vi "Time.vi"(8 "error in (no error)":errorcluster, 10 "Control In":T1={"I-O.lvclass"=refnum, "Gantry"=refnum, "Dispenser"="COM1"}, 11 "C4 Dispense in":refnum<class "Iterative Dispense.lvclass">) -> (0 "error out":errorcluster, 1 "Timing Data":i32[](array[numeric]), 2 "Control Out":T1={"I-O.lvclass"=refnum, "Gantry"=refnum, "Dispenser"="COM1"}, 3 "C4 Dispense out":refnum<class "Iterative Dispense.lvclass">)   [LabVIEW 2020, in "Iterative Dispense.lvclass"]
uses:
  Iterative Dispense.lvclass
  C:/Users/HEP/Documents/GitHub/UCSB-Gantry-HEP/Classes/Routine/Dispense/Dispense.lvclass
  Controller/Controllers.ctl
  Controller/I-O/I-O.lvclass
  C:/Program Files (x86)/Aerotech/A3200/LabVIEW/2010/Bin/Aerotech.A3200.dll
  Program Files (x86)/Aerotech/A3200/LabVIEW/2010/Bin/Aerotech.A3200.dll
  Iterative Dispense.lvclass/Iterative Dispense.ctl
  Controller/Motion/Motion.lvclass
  Controller/Motion/A3200/A3200.lvclass
  Controller/Controller.lvclass
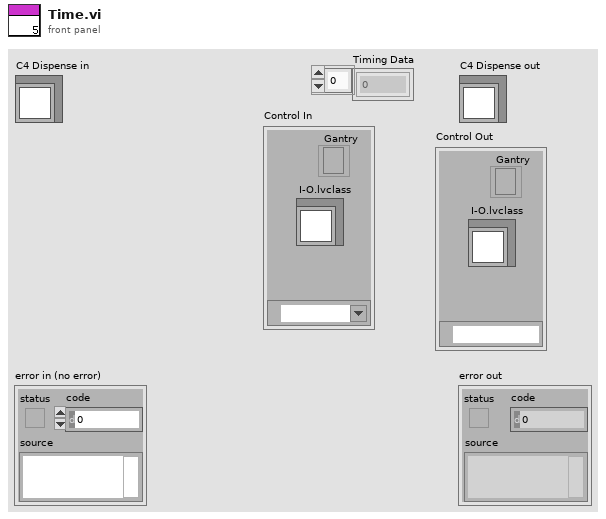
[diagram p1: front panel]
types:
  T1 = typedef "Controller.lvclass/Controllers.ctl" = cluster{"I-O.lvclass":refnum<class "I-O.lvclass">, "Gantry":refnum<k24>, "Dispenser":refnum<visa-resource-name>}
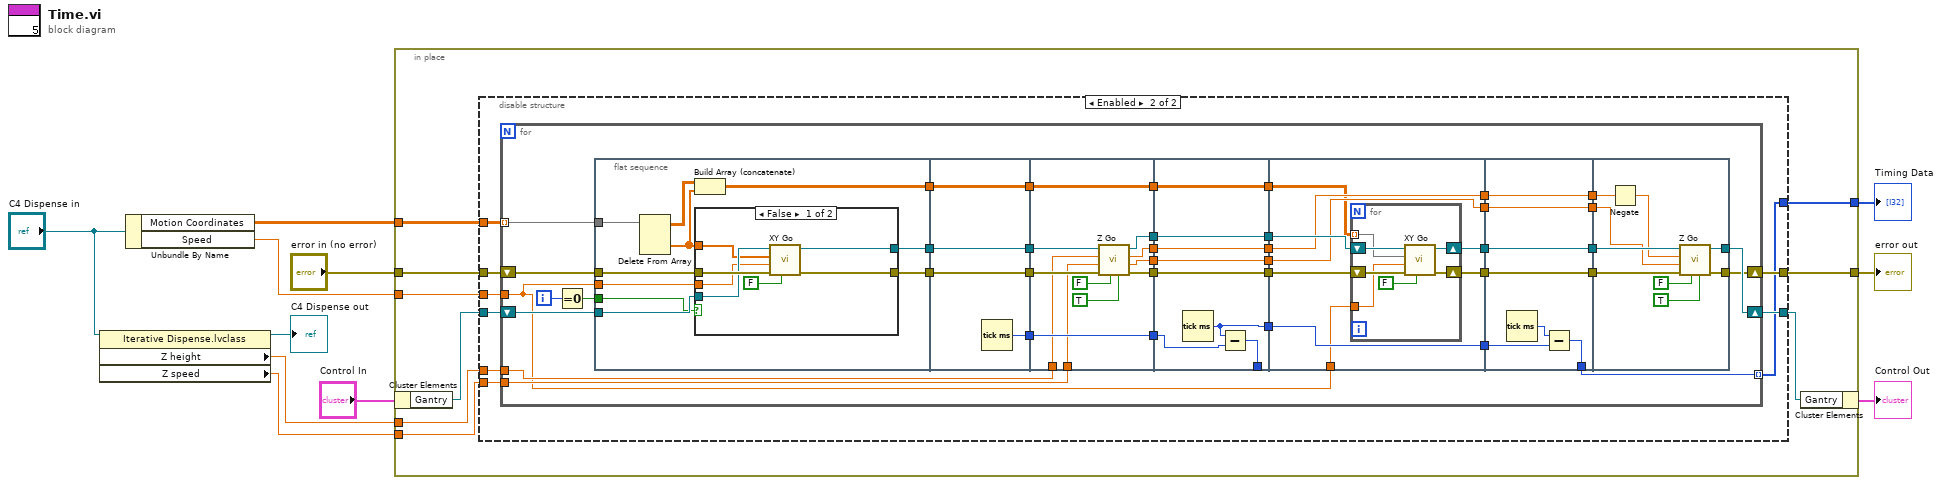
[diagram p0: block diagram]
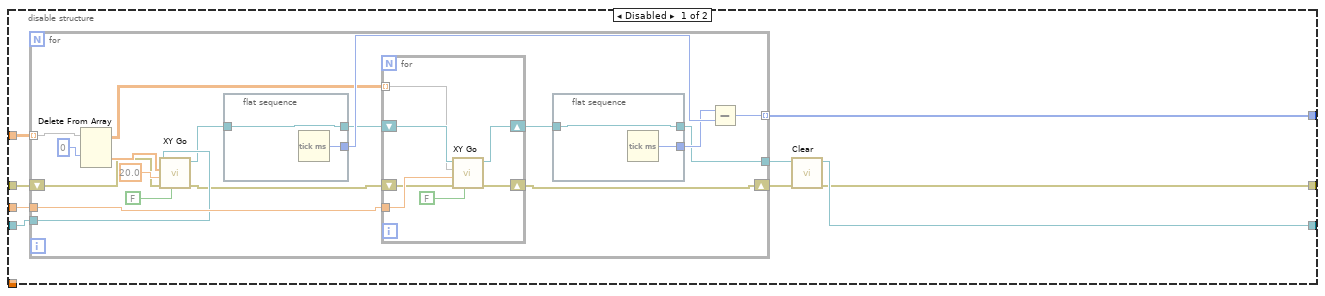
[diagram p2: hidden frame]
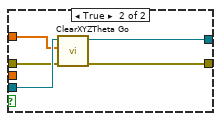
[diagram p3: hidden frame]
diagram:
  n1 = property class="Iterative Dispense.lvclass"(reference="C4 Dispense in") -> (reference out=→"C4 Dispense out":refnum<class "Iterative Dispense.lvclass">, "Z height"=w1:dbl, "Z speed"=w2:dbl)  [unwired: 1 in, 1 out]
  n2 = Unbundle By Name("C4 Dispense in") -> ("Motion Coordinates"=w11:dbl[][][], "Speed"=w7:dbl)
  n3 = in-place {
    in-place-border: w11 -> [w20]
    in-place-border: [w19] -> w10
    in-place-border: w7 -> [w18]
    in-place-border: "error in (no error)" -> [w15]
    in-place-border: [w14] -> w5
    in-place-border: w2 -> [w13]
    in-place-border: w1 -> [w12]
    n4 = in-place-cluster #1("Control In") -> ("Gantry"=w17:refnum<k24>)
    n5 = disable-structure shown="Enabled" {
      disable-tunnel: w20 -> [w29 w67]
      disable-tunnel: [w28 w59] -> w19
      disable-tunnel: w18 -> [w27 w62]
      disable-tunnel: w17 -> [w26 w66]
      disable-tunnel: [w25 w61] -> w16
      disable-tunnel: w15 -> [w23 w65]
      disable-tunnel: [w21 w60] -> w14
      disable-tunnel: w13 -> [_ w64]
      disable-tunnel: w12 -> [_ w63]
      frame Disabled {
        n6 = for {
          tunnel: [w45] -> w28 mode=indexing
          tunnel: w29 -> [w42] mode=indexing
          tunnel: w27 -> [w41]
          tunnel: w26 -> [w39]
          tunnel: [w36] -> w24
          shift-right: [w31] -> w22
          shift-left: w23 -> [w33]
          n7 = Delete From Array(array=w42, index (row)=0) -> (deleted portion=w35:dbl[], array with subset deleted=w44:dbl[][])  [unwired: 2 in]
          n8 = call "XY Go.vi"("return immediately"=FALSE, "error in (no error)"=w33, "Speed"=20.0, "XY In"=w35, "Gantry In"=w39) -> ("error out"=w32:errorcluster, "Gantry Out"=w38:refnum<k24>)  [unwired: 4 in, 1 out]
          n9 = flat-sequence {
            tunnel: [w51] -> w47
            tunnel: w38 -> [w50]
            tunnel: [w50] -> w37
            frame #0 {
              n10 = Tick Count (ms)() -> (millisecond timer value=w51:u32)
            }
          }
          n11 = for {
            tunnel: w44 -> [w56] mode=indexing
            tunnel: w41 -> [w55]
            shift-right: [w57] -> w40
            shift-left: w37 -> [w58]
            shift-right: [w53] -> w31
            shift-left: w32 -> [w54]
            n12 = call "XY Go.vi"("return immediately"=FALSE, "error in (no error)"=w54, "Speed"=w55, "XY In"=w56, "Gantry In"=w58) -> ("error out"=w53:errorcluster, "Gantry Out"=w57:refnum<k24>)  [unwired: 4 in, 1 out]
          }
          n13 = flat-sequence {
            tunnel: [w49] -> w46
            tunnel: [w48] -> w36
            tunnel: w40 -> [w48]
            frame #0 {
              n14 = Tick Count (ms)() -> (millisecond timer value=w49:u32)
            }
          }
          n15 = Subtract(x=w46, y=w47) -> (x-y=w45:u32)
        }
        n16 = call "Clear.vi"("error in (no error)"=w22, "Gantry In"=w24) -> ("error out"=w21:errorcluster, "Gantry Out"=w25:refnum<k24>)  [unwired: 8 in]
      }
      frame Enabled {
        n17 = for {
          tunnel: w67 -> [w81] mode=indexing
          tunnel: w64 -> [w79]
          tunnel: w63 -> [w78]
          tunnel: w62 -> [w68]
          tunnel: [w71] -> w59 mode=indexing
          shift-right: [w73] -> w61
          shift-left: w66 -> [w82]
          shift-right: [w72] -> w60
          shift-left: w65 -> [w80]
          i -> [w70]
          n18 = Equal To 0?(x=w70) -> (x = 0?=w69:bool)
          n19 = flat-sequence {
            tunnel: [w116] -> w106
            tunnel: [w115] -> w105
            tunnel: w82 -> [w114]
            tunnel: w81 -> [w113]
            tunnel: w80 -> [w112]
            tunnel: [w107] -> w74
            tunnel: w69 -> [w111]
            tunnel: w68 -> [w110]
            tunnel: w106 -> [w131]
            tunnel: [w131] -> w104
            tunnel: [w132] -> w103
            tunnel: [w130] -> w102
            tunnel: w105 -> [w130]
            tunnel: [w129] -> w75
            tunnel: w74 -> [w129]
            tunnel: w104 -> [w144]
            tunnel: [w143] -> w101
            tunnel: w103 -> [w143]
            tunnel: [w142] -> w100
            tunnel: [w141] -> w99
            tunnel: [w140] -> w98
            tunnel: w102 -> [w139]
            tunnel: [w138] -> w97
            tunnel: w79 -> [w135]
            tunnel: w78 -> [w134]
            tunnel: [w133] -> w76
            tunnel: w75 -> [w133]
            tunnel: w101 -> [w152]
            tunnel: [w151] -> _
            tunnel: [w150] -> w96
            tunnel: w100 -> [w150]
            tunnel: [w149] -> w95
            tunnel: [w148] -> w94
            tunnel: w99 -> [w148]
            tunnel: [w147] -> w93
            tunnel: w98 -> [w147]
            tunnel: w97 -> [w146]
            tunnel: [w146] -> w92
            tunnel: [w145] -> w77
            tunnel: w76 -> [w145]
            tunnel: w96 -> [w161]
            tunnel: [w160] -> w91
            tunnel: w95 -> [w160]
            tunnel: [w159] -> w90
            tunnel: [w158] -> w89
            tunnel: w94 -> [w158]
            tunnel: [w157] -> w88
            tunnel: w93 -> [w157]
            tunnel: w92 -> [w156]
            tunnel: [w155] -> w87
            tunnel: w77 -> [w154]
            tunnel: w68 -> [w153]
            tunnel: w91 -> [w174]
            tunnel: [w173] -> w86
            tunnel: w90 -> [w173]
            tunnel: [w172] -> w85
            tunnel: w89 -> [w172]
            tunnel: [w171] -> w84
            tunnel: w88 -> [w171]
            tunnel: [w170] -> w83
            tunnel: w87 -> [w170]
            tunnel: [w169] -> w71
            tunnel: w86 -> [w184]
            tunnel: w85 -> [w183]
            tunnel: w84 -> [w181]
            tunnel: [w180] -> w73
            tunnel: w83 -> [w179]
            tunnel: [w178] -> w72
            frame #0 {
              n20 = Delete From Array(array=w113) -> (deleted portion=w108:dbl[], array with subset deleted=w109:dbl[][])  [unwired: 3 in]
              n21 = Build Array (concatenate)(w109, w108) -> (w107:dbl[][])
              n22 = case shown="False" w111 {
                tunnel: [w123 w128] -> w116
                tunnel: [w122 w127] -> w115
                tunnel: w114 -> [w119 w126]
                tunnel: w108 -> [w118 w125]
                tunnel: w112 -> [w120 w124]
                tunnel: w110 -> [w117 _]
                frame False {
                  n23 = call "XY Go.vi"("return immediately"=FALSE, "error in (no error)"=w120, "Speed"=w117, "XY In"=w118, "Gantry In"=w119) -> ("error out"=w122:errorcluster, "Gantry Out"=w123:refnum<k24>)  [unwired: 4 in, 1 out]
                }
                frame True {
                  n24 = call "ClearXYZTheta Go.vi"("error in (no error)"=w124, "XYZTheta In"=w125, "Gantry In"=w126) -> ("error out"=w127:errorcluster, "Gantry Out"=w128:refnum<k24>)  [unwired: 6 in, 1 out]
                }
              }
            }
            frame #1 {
              n25 = Tick Count (ms)() -> (millisecond timer value=w132:u32)
            }
            frame #2 {
              n26 = call "Z Go.vi"("Increment"=TRUE, "Return Immediately"=FALSE, "error in (no error)"=w139, "Speed In"=w135, "Position In"=w134, "Gantry In"=w144) -> ("error out"=w138:errorcluster, "Speed Out"=w140:dbl, "Position Out"=w141:dbl, "Gantry Out"=w142:refnum<k24>)  [unwired: 2 in]
            }
            frame #3 {
              n27 = Tick Count (ms)() -> (millisecond timer value=w149:u32)
              n28 = Subtract(x=w149, y=w152) -> (x-y=w151:u32)
            }
            frame #4 {
              n29 = for {
                shift-right: [w167] -> w159
                shift-left: w161 -> [w168]
                shift-right: [w165] -> w155
                shift-left: w156 -> [w166]
                tunnel: w154 -> [w163] mode=indexing
                tunnel: w153 -> [w162]
                n30 = call "XY Go.vi"("return immediately"=FALSE, "error in (no error)"=w166, "Speed"=w162, "XY In"=w163, "Gantry In"=w168) -> ("error out"=w165:errorcluster, "Gantry Out"=w167:refnum<k24>)  [unwired: 4 in, 1 out]
              }
            }
            frame #5 {
              n31 = Tick Count (ms)() -> (millisecond timer value=w175:u32)
              n32 = Subtract(x=w175, y=w174) -> (x-y=w169:u32)
            }
            frame #6 {
              n33 = Negate(x=w183) -> (-x=w182:dbl)
              n34 = call "Z Go.vi"("Increment"=TRUE, "Return Immediately"=FALSE, "error in (no error)"=w179, "Speed In"=w181, "Position In"=w182, "Gantry In"=w184) -> ("error out"=w178:errorcluster, "Gantry Out"=w180:refnum<k24>)  [unwired: 2 in, 2 out]
            }
          }
        }
      }
    }
    n35 = in-place-cluster #1("Gantry"=w16) -> (→"Control Out":T1)
  }
  "error out" <- w5
  "Timing Data" <- w10
